vi "Simulation Robot Open.vi"(8 "error in (no error)":errorcluster, 11 "RoboSimIDs":T1) -> (0 "error out":errorcluster, 2 "initial position":sgl[](array[numeric]), 3 "Robot":T3)   [LabVIEW 2014]
doc: "Begins a simulation of the Cal Climber."
uses:
  Multi Bot Code/RobotData.ctl
  <instrlib>/DC Motor Controller/HAIOL/DC Motor Controller.lvclass
  Multi Bot Code/SensorType.ctl
  SimulationIDs.ctl
  <vilib>/Robotics/Simulator/Engine/ctl/DeviceID.ctl
  <vilib>/Robotics/Simulator/Interface/Simulator References/Get Robot Body Reference.vi
  <vilib>/Robotics/Simulator/Interface/Simulator References/Get Sensor Reference.vi
  <vilib>/robotics/Simulator/NI_Robotics_Simulator.lvlib
  <resource>/objmgr/LVODE.rc
  <instrlib>/DC Motor Controller/HAIOL/Simulator/DC Motor Controller Simulator.lvclass
panel:
  out "SensorType":T2 items=["BumperSensor"=1, "DistanceSensor"=2, "AccelerometerSensor"=3, "Wall Sensor"=4, "Unknown"=0]
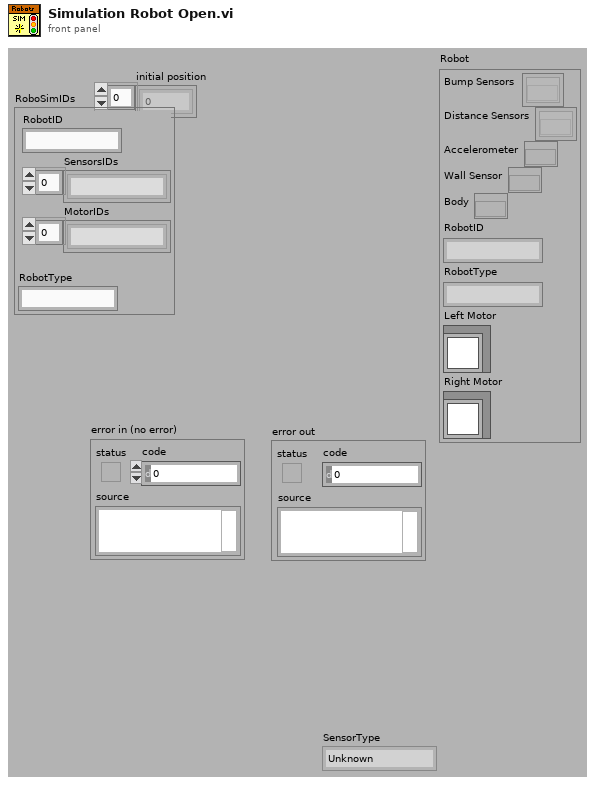
[diagram p1: front panel]
types:
  T1 = typedef "SimulationIDs.ctl" = cluster{"RobotID":string, "SensorsIDs":string[], "MotorIDs":string[], "RobotType":string}
  T2 = typedef "SensorType.ctl" = u16
  T3 = typedef "RobotData.ctl" = cluster{"Bump Sensors":refnum<k20>[], "Distance Sensors":refnum<k20>[], "Accelerometer":refnum<k20>, "Wall Sensor":refnum<k20>, "Body":refnum<k20>, "RobotID":string, "RobotType":string, "Left Motor":refnum<class "DC Motor Controller.lvclass">, "Right Motor":refnum<class "DC Motor Controller.lvclass">}
  T4 = typedef "NI_Robotics_Simulator.lvlib/DeviceID.ctl" = cluster{"robot ID":string, "sensor/actuator ID":string}
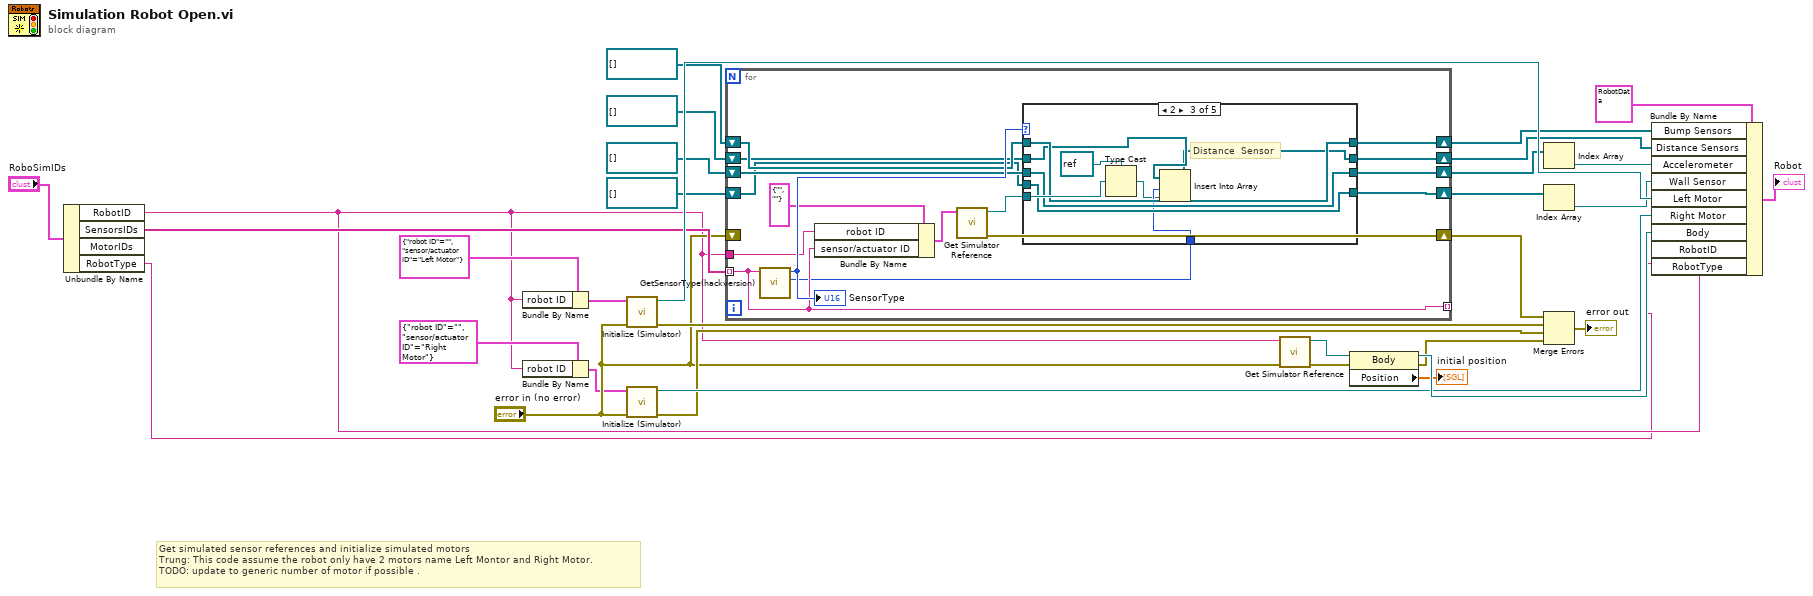
[diagram p0: block diagram]
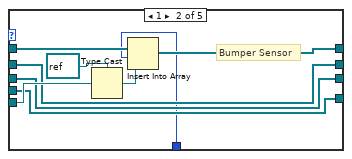
[diagram p3: hidden frame]
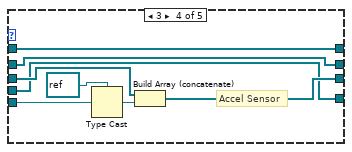
[diagram p4: hidden frame]
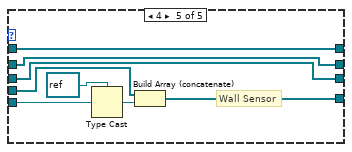
[diagram p5: hidden frame]
diagram:
  # "Get simulated sensor references and initialize simulated motors\nTrung: This code assume the robot only have 2 motors name Left Montor and Right Motor.\nTODO: update to generic number of motor if possible ."
  n1 = Unbundle By Name("RoboSimIDs") -> ("RobotID"=w2:string, "SensorsIDs"=w13:string[], "RobotType"=w1:string)  [unwired: 1 out]
  n2 = Bundle By Name(cluster=T4 {"robot ID"="", "sensor/actuator ID"="Left Motor"} ("Device ID"), "robot ID"=w2) -> (w20:T4)
  n3 = Bundle By Name(cluster=T4 {"robot ID"="", "sensor/actuator ID"="Right Motor"} ("Device ID"), "robot ID"=w2) -> (w3:T4)
  n4 = call <instrlib>:"Initialize (Simulator).vi"("error in (no error)"="error in (no error)", "Device ID"=w20) -> ("error out"=w28:errorcluster, "DC Motor Controller out"=w29:refnum<class "DC Motor Controller.lvclass">)  [unwired: 8 in]
  n5 = call <instrlib>:"Initialize (Simulator).vi"("error in (no error)"="error in (no error)", "Device ID"=w3) -> ("error out"=w26:errorcluster, "DC Motor Controller out"=w27:refnum<class "DC Motor Controller.lvclass">)  [unwired: 8 in]
  n6 = for {
    shift-right: [w46] -> w8
    shift-left: refnum<k20>[] [] ("Bump Sensors") -> [w47]
    shift-right: [w44] -> w7
    shift-left: refnum<k20>[] [] ("Distance Sensors") -> [w45]
    shift-right: [w42] -> w10
    shift-left: refnum<k20>[] [] ("Bump Sensors") -> [w43]
    shift-right: [w40] -> w12
    shift-left: refnum<k20>[] [] ("Bump Sensors") -> [w41]
    tunnel: [w34] -> _ mode=indexing
    tunnel: w13 -> [w34] mode=indexing
    tunnel: w2 -> [w39]
    shift-right: [w35] -> w5
    shift-left: "error in (no error)" -> [_]
    n7 = call "GetSensorType(hackversion).vi"("Accessors:ID"=w34) -> ("offset"=w33:i32, "SensorType"=w48:T2)  [unwired: 9 in]
    "SensorType" <- w48
    n8 = Bundle By Name(cluster=T4 {"robot ID"="", "sensor/actuator ID"=""} ("Device ID"), "robot ID"=w39, "sensor/actuator ID"=w34) -> (w38:T4)
    n9 = call-poly <vilib>:"Get Simulator Reference.vi"("device ID"=w38) -> ("error out"=w35:errorcluster, "sensor ref"=w36:refnum<k20>)  [unwired: 9 in]
    n10 = case shown="2" w48 {
      tunnel: w36 -> [_ w60 w69 w77 w85]
      tunnel: [w52 w55 w68 w76 w84] -> w46
      tunnel: w47 -> [w52 w56 w68 w76 w84]
      tunnel: [w51 w59 w62 w75 w83] -> w44
      tunnel: w45 -> [w51 w59 w65 w75 w83]
      tunnel: [w50 w58 w67 w72 w79] -> w42
      tunnel: w43 -> [w50 w58 w67 w74 w79]
      tunnel: w41 -> [w49 w57 w66 w71 w81]
      tunnel: [w49 w57 w66 w71 w80] -> w40
      tunnel: w33 -> [_ w53 w64 _ _]
      frame 0, Default {
      }
      frame 1 {
        # "Bumper Sensor"
        n11 = Type Cast(type=refnum<k20> refnum ("LVODE Refnum"), x=w60) -> (*(type *) &x=w54:refnum<k20>)
        n12 = Insert Into Array(array=w56, index=w53, new element=w54) -> (w55:refnum<k20>[])
      }
      frame 2 {
        # "Distance  Sensor"
        n13 = Type Cast(type=refnum<k20> refnum ("LVODE Refnum"), x=w69) -> (*(type *) &x=w63:refnum<k20>)
        n14 = Insert Into Array(array=w65, index=w64, new element=w63) -> (w62:refnum<k20>[])
      }
      frame 3 {
        # "Accel Sensor"
        n15 = Type Cast(type=refnum<k20> refnum ("LVODE Refnum"), x=w77) -> (*(type *) &x=w73:refnum<k20>)
        n16 = Build Array (concatenate)(w74, w73) -> (w72:refnum<k20>[])
      }
      frame 4 {
        # "Wall Sensor"
        n17 = Type Cast(type=refnum<k20> refnum ("LVODE Refnum"), x=w85) -> (*(type *) &x=w82:refnum<k20>)
        n18 = Build Array (concatenate)(w81, w82) -> (w80:refnum<k20>[])
      }
    }
  }
  n19 = call-poly <vilib>:"Get Simulator Reference.vi"("error in (no error)"="error in (no error)", "robot ID"=w2) -> ("error out"=w24:errorcluster, "robot body ref"=w25:refnum<k20>)  [unwired: 8 in]
  n20 = property class="Body"(reference=w25, error in=w24) -> (reference out=w32:refnum<k20>, error out=w23:errorcluster, "Position"=→"initial position":sgl[])
  n21 = Index Array(array=w10) -> (element=w9:refnum<k20>)  [unwired: 1 in]
  n22 = Index Array(array=w12) -> (element=w11:refnum<k20>)  [unwired: 1 in]
  n23 = Merge Errors(w5, w28, w26, w23) -> (→"error out":errorcluster)
  n24 = Bundle By Name(cluster=T3 {"Bump Sensors"=[], "Distance Sensors"=[], "Accelerometer"=refnum, "Wall Sensor"=refnum, "Body"=refnum, "RobotID"="", "RobotType"="", "Left Motor"=refnum, "Right Motor"=refnum} ("Robot"), "Bump Sensors"=w8, "Distance Sensors"=w7, "Accelerometer"=w9, "Wall Sensor"=w11, "Left Motor"=w29, "Right Motor"=w27, "Body"=w32, "RobotID"=w2, "RobotType"=w1) -> (→"Robot":T3)
